vi "Dispenser Test.vi"() -> ()   [LabVIEW 2020]
uses:
  Drivers/EFD Ultimus V/EFD Ultimus V.lvlib
panel:
  in  "pressure(psi)":i32
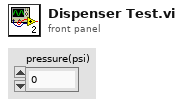
[diagram p1: front panel]
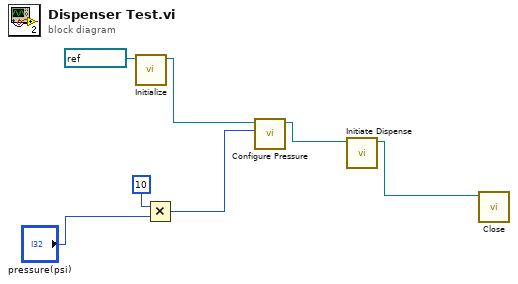
[diagram p0: block diagram]
diagram:
  n1 = call "Initialize.vi"("VISA resource name"=refnum<visa-resource-name> "COM1") -> ("VISA resource name out"=w6:refnum<visa-resource-name>)  [unwired: 8 in, 1 out]
  n2 = Multiply(x=10, y="pressure(psi)") -> (x*y=w3:i32)
  n3 = call "Configure Pressure.vi"("Pressure Setting (0000)"=w3, "VISA resource name"=w6) -> ("VISA resource name out"=w2:refnum<visa-resource-name>)  [unwired: 8 in, 1 out]
  n4 = call "Initiate Dispense.vi"("VISA resource name"=w2) -> ("VISA resource name out"=w1:refnum<visa-resource-name>)  [unwired: 9 in, 1 out]
  n5 = call "Close.vi"("VISA resource name"=w1) -> ()  [unwired: 10 in, 1 out]
